vi "Teleop.vi"(10 "Match Info":T1={"Autonomous Elapsed Seconds"=0.0, "TeleOp Elapsed Seconds"=0.0, "Disabled Elapsed Seconds"=0.0, "Visited Autonomous"=FALSE, "Visited TeleOp"=FALSE, "Visited Disabled"=FALSE, "Autonomous Settings"={"Autonomous Style"=enum."Independent", "VI Refnum"=refnum}}, 11 "Call Context":T2) -> ()   [LabVIEW 2011]
doc: "This VI is called for each TeleOp packet received from the DS where the robot is not disabled. It is often used to read from the joysticks and update I/O or to update setpoints for timed control loops. It should complete and return within 20 milliseconds or it may miss DS packets."
uses:
  <vilib>/Rock Robotics/WPI/DriverStation/WPI_DriverStationDerivedRobotMode.ctl
  <vilib>/Rock Robotics/WPI/DriverStation/WPI_DriverStationMatch Info.ctl
  Robot Global Data.vi
  Global.vi
  Pivot Drive.lvlib
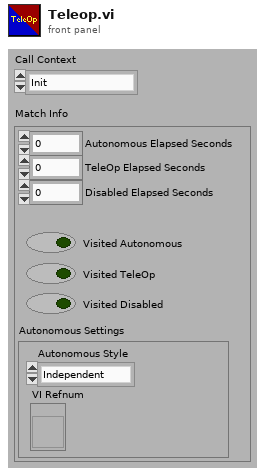
[diagram p1: front panel]
types:
  T1 = typedef "WPI_DriverStationMatch Info.ctl" = cluster{"Autonomous Elapsed Seconds":dbl, "TeleOp Elapsed Seconds":dbl, "Disabled Elapsed Seconds":dbl, "Visited Autonomous":bool, "Visited TeleOp":bool, "Visited Disabled":bool, "Autonomous Settings":cluster{"Autonomous Style":enum16{"Iterative", "Independent"}, "VI Refnum":refnum<vi>}}
  T2 = typedef "WPI_DriverStationDerivedRobotMode.ctl" = enum16{"Init", "Execute", "Stop"}
  T3 = typedef "WPI_JoystickDevRef.ctl" = cluster{"Device":T4}
  T4 = typedef "WPI_JoystickDeviceEnum.ctl" = enum16{"USB 1", "USB 2", "USB 3", "USB 4", "Kinect 1", "Kinect 2"}
  T5 = typedef "WPI_AnalogChannelDevRef.ctl" = cluster{"DevStatus":errorcluster, "Analog Module":T6, "Analog Channel":T7}
  T6 = typedef "FPGA_TypedefAnalogModule.ctl" = enum16{"Analog Module 1", "Analog Module 2"}
  T7 = typedef "FPGA_AIChannel.ctl" = enum8{"AI 1", "AI 2", "AI 3", "AI 4", "AI 5", "AI 6", "AI 7", "AI 8", "Invalid"}
  T8 = typedef "WPI_JoystickButtonState.ctl" = cluster{"Button 1":bool, "Button 2":bool, "Button 3":bool, "Button 4":bool, "Button 5":bool, "Button 6":bool, "Button 7":bool, "Button 8":bool, "Button 9":bool, "Button 10":bool, "Button 11":bool, "Button 12":bool}
  T9 = cluster{"axis 1 (x)":dbl, "axis 2 (y)":dbl, "axis 3 (throttle)":dbl, "axis 4":dbl, "axis 5":dbl, "axis 6":dbl}
  T10 = typedef "WPI_RobotDriveDevRef.ctl" = cluster{"DevStatus":errorcluster, "Motors[]":T11[], "Square Inputs":bool, "Max Output":dbl, "Isochronous":bool}
  T11 = typedef "WPI_MotorControlDeviceRef.ctl" = cluster{"DeviceStatus":errorcluster, "Type":enum16{"PWM", "CAN"}, "PWM":cluster{"Digital Module":T12, "PWM Channel":T13, "DeadBand":T14}, "CAN":cluster{"Device Number":u8, "Control Mode":T15, "Semaphore":T16, "Max Vout":dbl}, "Invert":bool, "TransformRef":T17, "InvTransformRef":T17}
  T12 = typedef "FPGA_TypedefDigitalModule.ctl" = enum16{"Digital Module 1", "Digital Module 2"}
  T13 = typedef "FPGA_DIOPWMChannel.ctl" = enum8{"PWM 1", "PWM 2", "PWM 3", "PWM 4", "PWM 5", "PWM 6", "PWM 7", "PWM 8", "PWM 9", "PWM 10", "Invalid"}
  T14 = typedef "WPI_PWMDeadband.ctl" = cluster{"Name":string, "maxPositivePwm":i32, "minPositivePwm":i32, "centerPwm":i32, "maxNegativePwm":i32, "minNegativePwm":i32, "angularRange":u16}
  T15 = typedef "WPI_CANJaguar_ControlMode.ctl" = enum8{"Percent VBus", "Current", "Speed", "Position", "Voltage"}
  T16 = typedef "Semaphore RefNum" = refnum<k1>
  T17 = typedef "WPI_PWMTransform_ConPane.ctl" = refnum<vi>
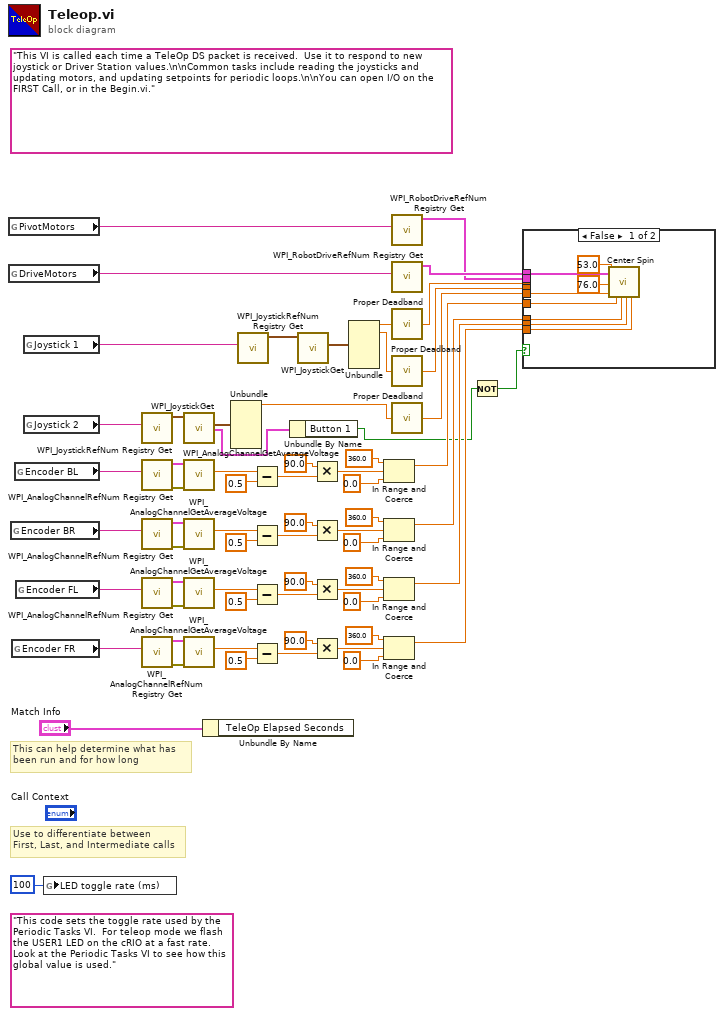
[diagram p0: block diagram]
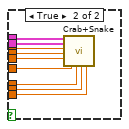
[diagram p2: hidden frame]
diagram:
  (unwired) "This code sets the toggle rate used by the Periodic Tasks VI.  For teleop mode we flash the USER1 LED on the cRIO at a fast rate.  Look at the Periodic Tasks VI to see how this global value is used."
  (unwired) "This VI is called each time a TeleOp DS packet is received.  Use it to respond to new joystick or Driver Station values.\n\nCommon tasks include reading the joysticks and updating motors, and updating setpoints for periodic loops.\n\nYou can open I/O on the FIRST Call, or in the Begin.vi."
  # "Use to differentiate between\nFirst, Last, and Intermediate calls"
  # "This can help determine what has\nbeen run and for how long"
  n1 = global read "Global.vi" "PivotMotors"() -> (w57:string)
  n2 = global read "Global.vi" "DriveMotors"() -> (w56:string)
  n3 = global read "Global.vi" "Encoder BR"() -> (w58:string)
  n4 = global read "Global.vi" "Encoder FR"() -> (w60:string)
  n5 = global read "Global.vi" "Encoder BL"() -> (w59:string)
  n6 = global read "Global.vi" "Encoder FL"() -> (w61:string)
  n7 = global read "Global.vi" "Joystick 1"() -> (w63:string)
  n8 = global read "Global.vi" "Joystick 2"() -> (w62:string)
  n9 = global write "Robot Global Data.vi" "LED toggle rate (ms)"(u32 100 ("LED ms toggle rate")) -> ()
  n10 = call <vilib>:"WPI_JoystickRefNum Registry Get.vi"("refnum name"=w62) -> ("JoystickDevRef"=w46:T3)  [unwired: 1 in, 9 out]
  n11 = call <vilib>:"WPI_AnalogChannelRefNum Registry Get.vi"("refnum name"=w59) -> ("error out"=w50:errorcluster, "AIDeviceRef"=w51:T5)  [unwired: 1 in, 8 out]
  n12 = call <vilib>:"WPI_AnalogChannelRefNum Registry Get.vi"("refnum name"=w58) -> ("error out"=w48:errorcluster, "AIDeviceRef"=w49:T5)  [unwired: 1 in, 8 out]
  n13 = call <vilib>:"WPI_AnalogChannelRefNum Registry Get.vi"("refnum name"=w61) -> ("error out"=w52:errorcluster, "AIDeviceRef"=w53:T5)  [unwired: 1 in, 8 out]
  n14 = call <vilib>:"WPI_AnalogChannelRefNum Registry Get.vi"("refnum name"=w60) -> ("error out"=w54:errorcluster, "AIDeviceRef"=w55:T5)  [unwired: 1 in, 8 out]
  n15 = call <vilib>:"WPI_JoystickGet.vi"("JoystickDevRef"=w46) -> ("Buttons"=w3:T8, "Axes"=w44:T9)  [unwired: 1 in, 4 out]
  n16 = call <vilib>:"WPI_AnalogChannelGetAverageVoltage.vi"("error in (no error)"=w50, "AIDeviceRef"=w51) -> ("Voltage"=w28:dbl)  [unwired: 9 out]
  n17 = call <vilib>:"WPI_AnalogChannelGetAverageVoltage.vi"("error in (no error)"=w48, "AIDeviceRef"=w49) -> ("Voltage"=w32:dbl)  [unwired: 9 out]
  n18 = call <vilib>:"WPI_AnalogChannelGetAverageVoltage.vi"("error in (no error)"=w52, "AIDeviceRef"=w53) -> ("Voltage"=w36:dbl)  [unwired: 9 out]
  n19 = call <vilib>:"WPI_AnalogChannelGetAverageVoltage.vi"("error in (no error)"=w54, "AIDeviceRef"=w55) -> ("Voltage"=w40:dbl)  [unwired: 9 out]
  n20 = Unbundle By Name("Match Info") -> ()  [unwired: 1 out]
  n21 = Unbundle(w44) -> ("axis 1 (x)"=w23:dbl)  [unwired: 5 out]
  n22 = call <vilib>:"WPI_JoystickRefNum Registry Get.vi"("refnum name"=w63) -> ("JoystickDevRef"=w47:T3)  [unwired: 1 in, 9 out]
  n23 = Subtract(x=w28, y=0.5) -> (x-y=w29:dbl)
  n24 = Subtract(x=w32, y=0.5) -> (x-y=w33:dbl)
  n25 = Subtract(x=w36, y=0.5) -> (x-y=w39:dbl)
  n26 = Subtract(x=w40, y=0.5) -> (x-y=w43:dbl)
  n27 = Unbundle By Name(w3) -> ("Button 1"=w2:bool)
  n28 = call <vilib>:"WPI_JoystickGet.vi"("JoystickDevRef"=w47) -> ("Axes"=w45:T9)  [unwired: 1 in, 5 out]
  n29 = Multiply(x=90.0, y=w29) -> (x*y=w21:dbl)
  n30 = Multiply(x=90.0, y=w33) -> (x*y=w16:dbl)
  n31 = Multiply(x=90.0, y=w39) -> (x*y=w13:dbl)
  n32 = Multiply(x=90.0, y=w43) -> (x*y=w10:dbl)
  n33 = Unbundle(w45) -> ("axis 1 (x)"=w26:dbl, "axis 2 (y)"=w25:dbl)  [unwired: 4 out]
  n34 = In Range and Coerce(upper limit=360.0, x=w21, lower limit=0.0 ("upper limit")) -> (coerced(x)=w9:dbl)  [unwired: 1 out]
  n35 = In Range and Coerce(upper limit=360.0, x=w16, lower limit=0.0 ("upper limit")) -> (coerced(x)=w8:dbl)  [unwired: 1 out]
  n36 = In Range and Coerce(upper limit=360.0, x=w13, lower limit=0.0 ("upper limit")) -> (coerced(x)=w7:dbl)  [unwired: 1 out]
  n37 = In Range and Coerce(upper limit=360.0, x=w10, lower limit=0.0 ("upper limit")) -> (coerced(x)=w6:dbl)  [unwired: 1 out]
  n38 = call <vilib>:"WPI_RobotDriveRefNum Registry Get.vi"("refnum name"=w57) -> ("RobotDriveDevRef"=w4:T10)  [unwired: 1 in, 9 out]
  n39 = call <vilib>:"WPI_RobotDriveRefNum Registry Get.vi"("refnum name"=w56) -> ("RobotDriveDevRef"=w5:T10)  [unwired: 1 in, 9 out]
  n40 = call "Proper Deadband.vi"("Value"=w26) -> ("Deadbanded Value"=w27:dbl)
  n41 = call "Proper Deadband.vi"("Value"=w25) -> ("Deadbanded Value"=w24:dbl)
  n42 = call "Proper Deadband.vi"("Value"=w23) -> ("Deadbanded Value"=w22:dbl)
  n43 = Not(x=w2) -> (.not. x?=w1:bool)
  n44 = case shown="False" w1 {
    tunnel: w27 -> [_ w83]
    tunnel: w24 -> [_ w82]
    tunnel: w22 -> [w72 w81]
    tunnel: w9 -> [w71 w80]
    tunnel: w8 -> [w70 w79]
    tunnel: w7 -> [w69 w78]
    tunnel: w6 -> [w68 w77]
    tunnel: w5 -> [w74 w76]
    tunnel: w4 -> [w73 w75]
    frame False {
      n45 = call "Center Spin.vi"("RobotDriveDevRef"=w74, "RobotPivotDevRef"=w73, "Width"=53.0, "Legnth"=76.0, "Joystick axis"=w72, "Rear Left Current Pivot Angle"=w71, "Rear Right Current Pivot Angle"=w70, "Front Left Current Pivot Angle"=w69, "Front Right Current Pivot Angle"=w68) -> ()  [unwired: 8 in, 3 out]
    }
    frame True {
      n46 = call "Crab+Snake.vi"("RobotDriveDevRef"=w76, "RobotPivotDevRef"=w75, "Joystick 1 X"=w83, "Joystick 1 Y"=w82, "Joystick 2 X"=w81, "Rear Left Current Pivot Angle"=w80, "Rear Right Current Pivot Angle"=w79, "Front Left Current Pivot Angle"=w78, "Front Right Current Pivot Angle"=w77) -> ()  [unwired: 1 in, 10 out]
    }
  }
